vi "load cells.vi"() -> ()   [LabVIEW 2019]
doc: "The myRIO Project template acquires acceleration data from the onboard accelerometer and displays the changes of acceleration values in a waveform chart."
uses:
  <vilib>/myRIO/Instrument Drivers/Onboard IO/AI/typedefs/AI Reference.ctl
  <vilib>/myRIO/Common/Instrument Driver Framework/Utilities/typedefs/myRIO Generic Hardware Reference.ctl
  <vilib>/myRIO/Common/Instrument Driver Framework/Utilities/typedefs/Hardware Version Enum.ctl
  <vilib>/myRIO/Common/Instrument Driver Framework/Utilities/typedefs/myRIO v1.0 Reference.ctl
  <vilib>/myRIO/Common/Instrument Driver Framework/Utilities/typedefs/Generic FPGA Reference.ctl
  <vilib>/myRIO/Common/Instrument Driver Framework/myRIO v1.0/AI/typedefs/AI Channels List.ctl
  <vilib>/myRIO/Common/Instrument Driver Framework/myRIO v1.0/AI/typedefs/AI Channels Enum.ctl
  <vilib>/myRIO/Common/Instrument Driver Framework/Utilities/typedefs/Analog Scaling Constants List.ctl
  <vilib>/myRIO/Common/Instrument Driver Framework/Utilities/typedefs/Analog Scaling Constants.ctl
  <vilib>/userDefined/High Color/nirio_resource_hc.ctl
  <vilib>/myRIO/Instrument Drivers/Onboard IO/PWM/typedefs/PWM Reference.ctl
  <vilib>/myRIO/Common/Instrument Driver Framework/myRIO v1.0/PWM/typedefs/PWM Channels Enum.ctl
  <vilib>/myRIO/Instrument Drivers/Onboard IO/PWM/typedefs/PWM Configuration.ctl
  <vilib>/myRIO/Common/Instrument Driver Framework/Utilities/vis/Is FPGA Ref Available.vi
  <vilib>/myRIO/Common/Instrument Driver Framework/myRIO v1.0/AI/vis/myRIO v1.1 Open AI.vi
  <vilib>/myRIO/Instrument Drivers/Onboard IO/AI/vis/Read.vi
  <vilib>/myRIO/Common/Instrument Driver Framework/myRIO v1.0/PWM/vis/myRIO v1.1 Open PWM.vi
  <vilib>/myRIO/Common/Instrument Driver Framework/Utilities/vis/Validate Channels.vi
  <vilib>/myRIO/Common/Instrument Driver Framework/myRIO v1.0/AI/vis/myRIO v1.0 Reserve AI.vi
  <vilib>/myRIO/Common/Instrument Driver Framework/myRIO v1.0/PWM/vis/myRIO v1.0 Reserve PWM.vi
  <vilib>/myRIO/Common/Instrument Driver Framework/myRIO v1.0/PWM/vis/myRIO v1.0 Close PWM.vi
  <vilib>/myRIO/Common/Instrument Driver Framework/myRIO v1.0/AI/vis/myRIO v1.0 Build MUX Configuration AI.vi
  <vilib>/myRIO/Common/Instrument Driver Framework/myRIO v1.0/Resource Manager/vis/myRIO v1.0 Reserve Channel List.vi
  <vilib>/myRIO/Common/Instrument Driver Framework/myRIO v1.0/PWM/vis/myRIO v1.0 Build MUX Configuration PWM.vi
  <vilib>/myRIO/Common/Instrument Driver Framework/myRIO v1.0/PWM/vis/myRIO v1.0 Unreserve PWM.vi
  <vilib>/myRIO/Common/Instrument Driver Framework/myRIO v1.0/Resource Manager/vis/myRIO v1.0 Reserve Channel.vi
  <vilib>/myRIO/Common/Instrument Driver Framework/myRIO v1.0/Resource Manager/vis/myRIO v1.0 Unreserve Channel.vi
  <vilib>/myRIO/Common/Instrument Driver Framework/myRIO v1.0/Resource Manager/vis/myRIO v1.0 Create Configuration List.vi
  <vilib>/myRIO/Common/Instrument Driver Framework/myRIO v1.0/Resource Manager/vis/myRIO v1.0 Unreserve Channel List.vi
  <vilib>/myRIO/Common/Instrument Driver Framework/myRIO v1.0/Resource Manager/vis/myRIO v1.0 Build Mutex Name.vi
  <vilib>/Utility/VariantDataType/GetNumericInfo.vi
  <vilib>/Utility/error.llb/Error Cluster From Error Code.vi
  <vilib>/myRIO/Common/Instrument Driver Framework/myRIO v1.0/myRIO v1.1 Open.vi
  <vilib>/myRIO/Common/Instrument Driver Framework/myRIO v1.0/AI/vis/myRIO v1.0 Get Scaling Constants AI.vi
  <vilib>/myRIO/Common/Instrument Driver Framework/Utilities/vis/IO Manager.vi
  <vilib>/myRIO/Common/Instrument Driver Framework/Utilities/vis/Configuration Manager.vi
  <vilib>/myRIO/Common/Instrument Driver Framework/myRIO v1.0/myRIO v1.0 Close.vi
  <vilib>/myRIO/Common/Instrument Driver Framework/myRIO v1.0/AI/vis/myRIO v1.0 Read AI.vi
  <vilib>/myRIO/Common/Instrument Driver Framework/myRIO v1.0/Resource Manager/vis/myRIO v1.0 Configure IO.vi
  <vilib>/myRIO/Common/Instrument Driver Framework/myRIO v1.0/PWM/vis/myRIO v1.0 Write PWM.vi
  <vilib>/myRIO/Common/Instrument Driver Framework/myRIO v1.0/PWM/vis/myRIO v1.0 Shutdown PWM.vi
  <vilib>/myRIO/Express VI/Onboard IO/AI/AI Express VI.xnode
  <vilib>/myRIO/Instrument Drivers/Onboard IO/AI/vis/myRIO AI Open.xnode
  <vilib>/myRIO/Instrument Drivers/Onboard IO/PWM/vis/myRIO PWM Open.xnode
  <vilib>/Waveform/WDTFileIO.llb/ Write Waveform to File.vi
  <vilib>/myRIO/Instrument Drivers/Onboard IO/PWM/PWM.lvlib
  <vilib>/myRIO/Instrument Drivers/Onboard IO/AI/AI.lvlib
  <vilib>/ptbypt/NI_PtbyPt.lvlib
panel:
  out "Sum Right":dbl
  out "sum left":dbl
  out "a0":dbl format="%0.2f"
  out "appended array":dbl[](array[numeric])
  in  "cal1 3":dbl[](array[numeric])
  out "x*y 3":dbl[](array[numeric])
  out "Sensor Axial Right":T1(graph)
  out "Sensor Axial Left":T1(graph)
  in  "gain":dbl
  out "Sensor 12":dbl format="%0.2f"
  out "Sensor 10":dbl format="%0.2f"
  out "x*y 2":dbl[](array[numeric])
  in  "cal1 2":dbl[](array[numeric])
  out "Right cp2":cluster{dbl[], dbl[]}(graph)
  out "CENTER OF PRESSURE RIGHT BELT 3":dbl(graph)
  out "Sensor 8":dbl format="%0.5f"
  out "Sensor 7":dbl format="%0.5f"
  out "Sensor 6":dbl format="%0.5f"
  out "Sensor 5":dbl format="%0.5f"
  out "Sensor Rear Rigth":T1(graph)
  out "Sensor Rear Left":T1(graph)
  out "Sensor Front Right":T1(graph)
  out "Sensor Front  Left":T1(graph)
  out "RIGHT BELT SENSORS IN ONE PLOT 2":T2(graph)
  out "error out 7":errorcluster
  in  "error in 6":errorcluster
  out "error out 6":errorcluster
  in  "STOP RIGHT MOTOR":bool
  in  "RIGHT MOTOR DUTY CYCLE":dbl(slide)=50.00000000000001 scale=0.0..100.0
  out "error out 4":errorcluster
  in  "STOP LEFT MOTOR":bool
  in  "LEFT MOTOR DUTY CYCLE":dbl(slide)=50.00000000000001 scale=0.0..100.0
  in  "Stop Button":bool
  in  "ZERO ALL SENSORS":bool
  out "x*y":dbl[](array[numeric])
  in  "cal1":dbl[](array[numeric])
  out "Left cp1":cluster{dbl[], dbl[]}(graph)
  out "CENTER OF PRESSURE LEFT BELT 2":dbl(graph)
  out "dt":u32(graph)
  out "Sensor 4":dbl format="%0.5f"
  out "Sensor 3":dbl format="%0.5f"
  out "Sensor 2":dbl format="%0.5f"
  out "Sensor 1":dbl=0.0038137989155123176 format="%0.5f"
  out "Sensor Rear Rigth":T1(graph)
  out "Sensor Rear Left":T1(graph)
  out "Sensor Front Right":T1(graph)
  out "Sensor Front  Left":T1(graph)
  out "LEFT BELT SENSORS IN ONE PLOT":T2(graph)
  out "error out 5":errorcluster
  in  "error in 5":errorcluster
  # "Calibration Left"
  # "Calibration Right"
  # "Calibration Axial"
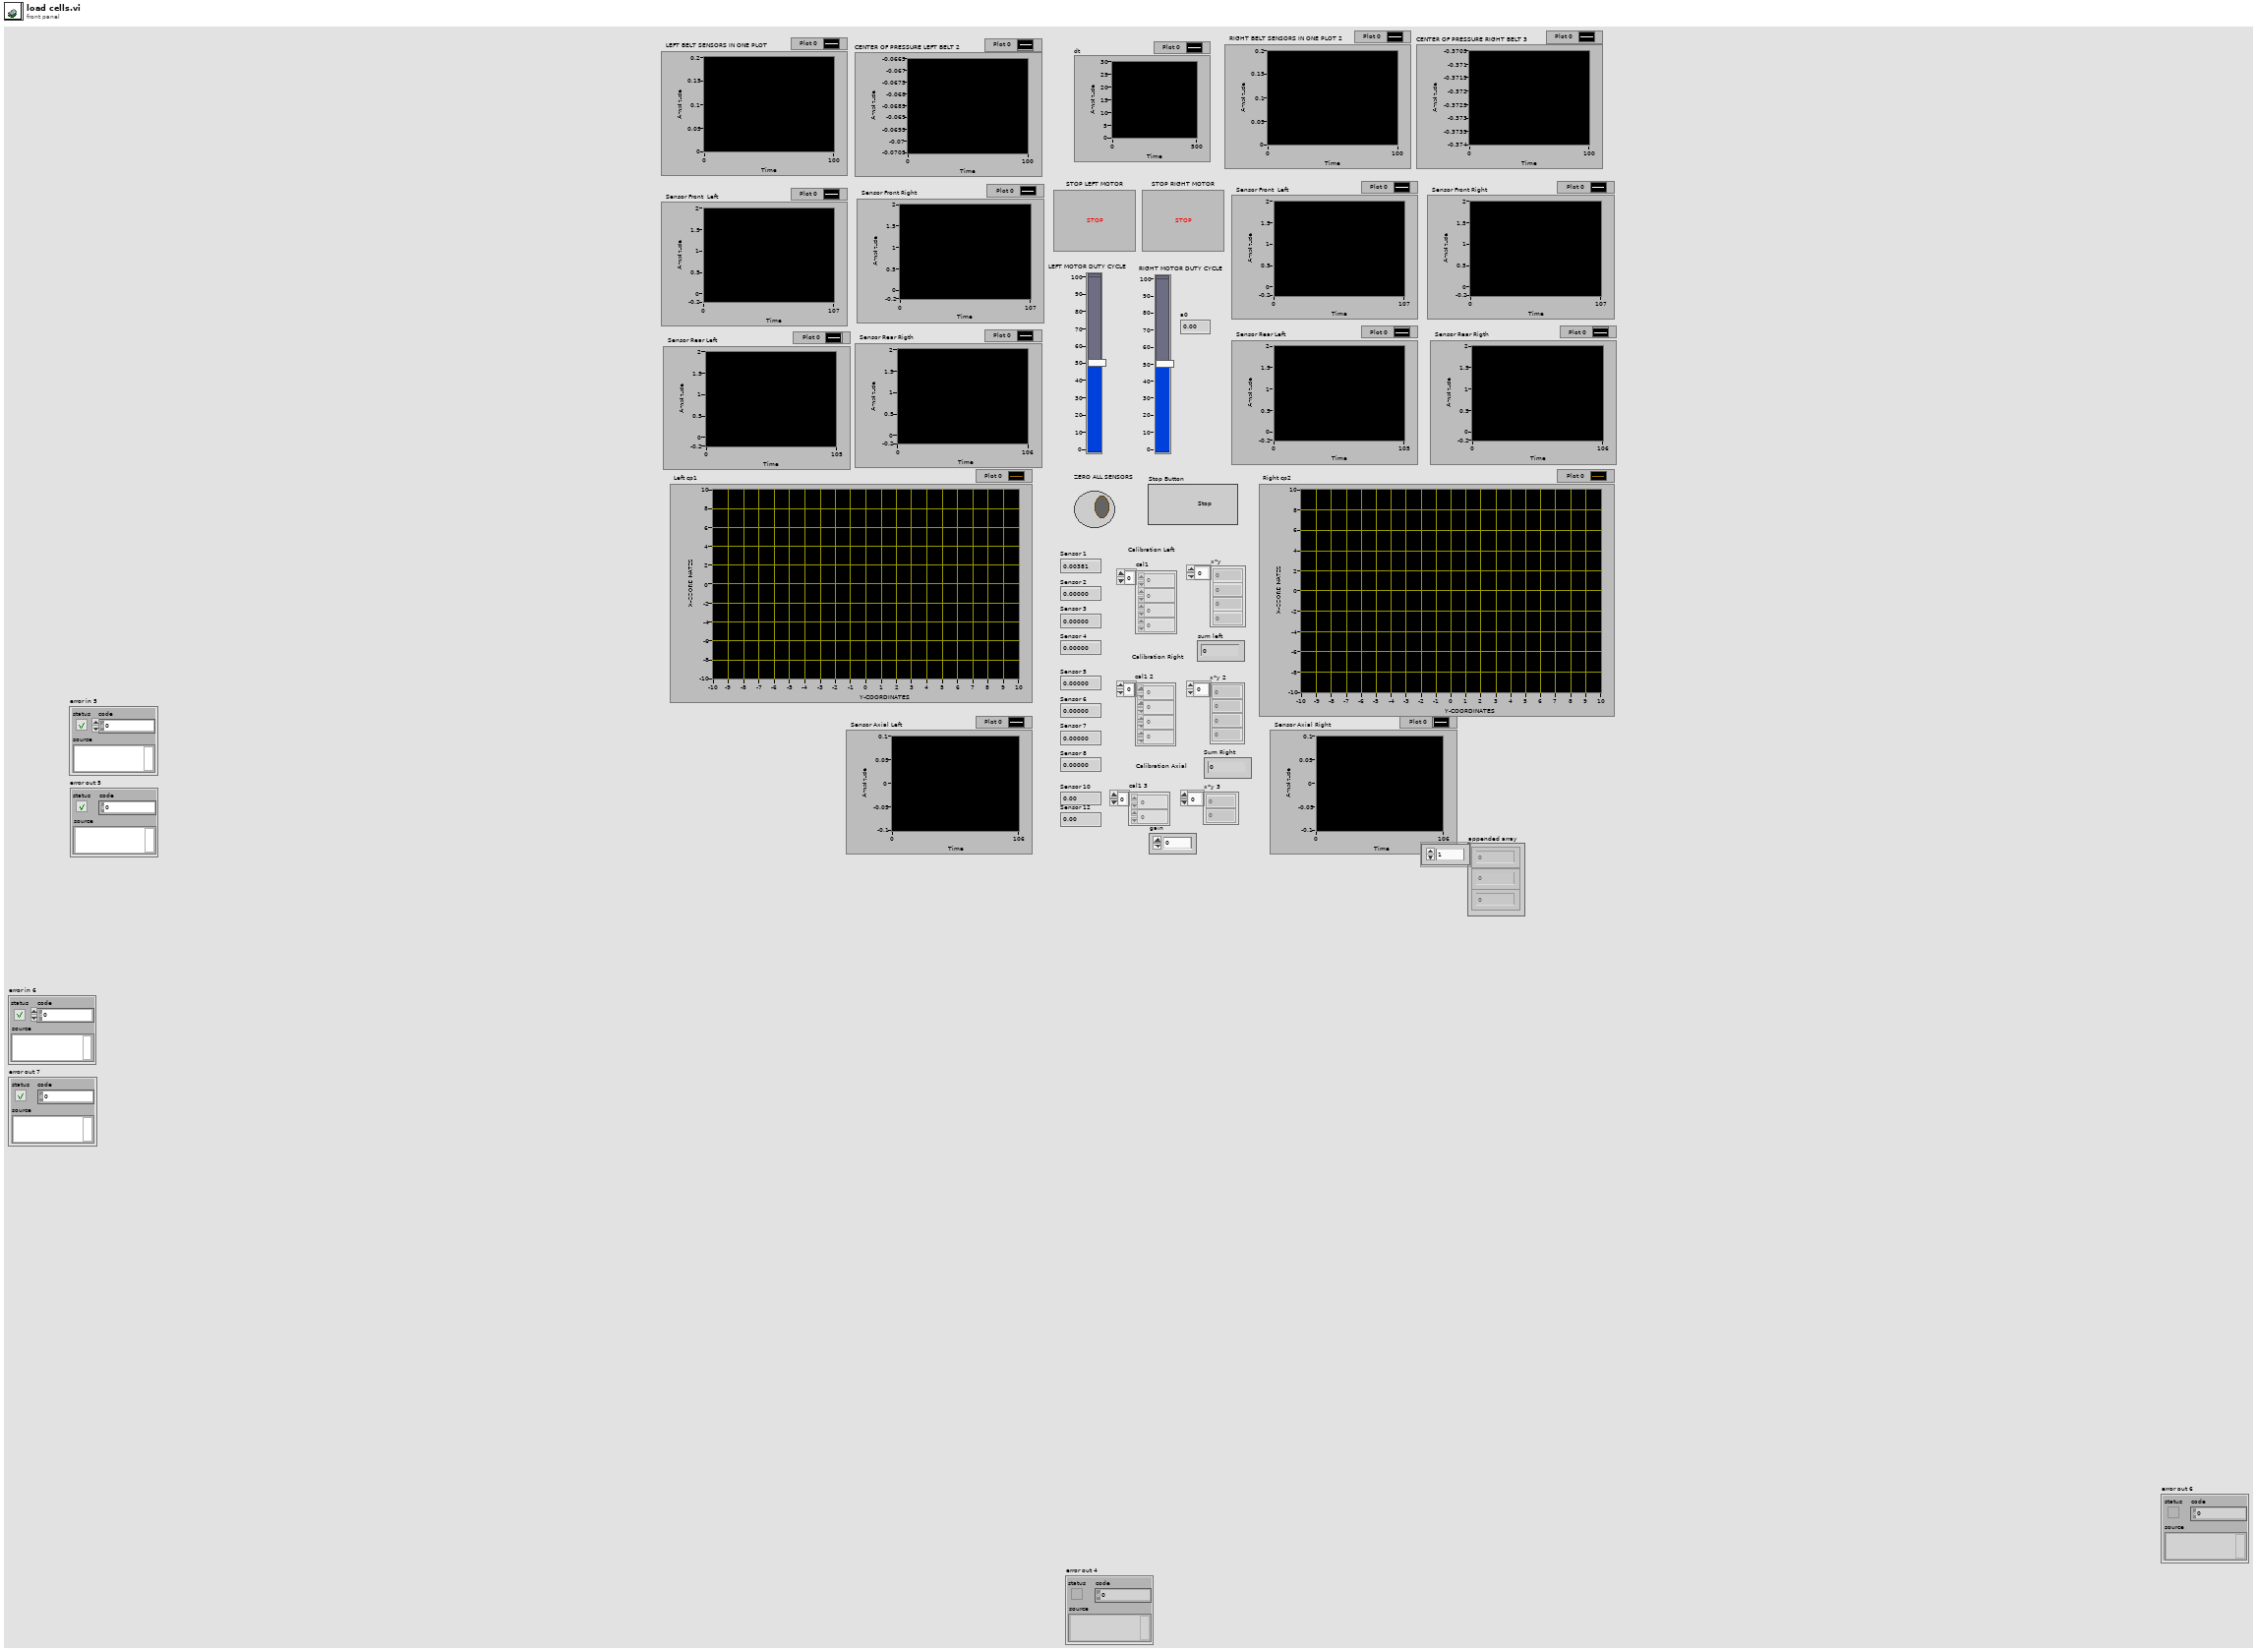
[diagram p1: front panel]
types:
  T1 = cluster{"Filtered x":dbl, "Sensor 1 (A/AI0 (Pin 3))":dbl}
  T2 = cluster{"Sensor 1 (A/AI0 (Pin 3))":dbl, "Sensor 2 (A/AI1 (Pin 5))":dbl, "Sensor 3 (A/AI2 (Pin 7))":dbl, "Sensor 4 (A/AI3 (Pin 9))":dbl}
  T3 = typedef "PWM.lvlib/PWM Reference.ctl" = cluster{"myRIO Reference":T4, "PWM Channels Enum":T8, "PWM Configuration":T9}
  T4 = typedef "myRIO Generic Hardware Reference.ctl" = cluster{"myRIO Model":T5, "myRIO Hardware Reference":T6}
  T5 = typedef "Hardware Version Enum.ctl" = enum16{"Unknown", "myRIO-1900", "myRIO-1950", "roboRIO", "NI ELVIS RIO CM", "ELVIS III"}
  T6 = typedef "myRIO v1.0 Reference.ctl" = cluster{"Generic FPGA Reference":T7, "Allow multiple opens":bool}
  T7 = typedef "Generic FPGA Reference.ctl" = refnum<k20>
  T8 = typedef "PWM Channels Enum.ctl" = enum16{"Not Connected", "C/PWM0", "C/PWM1", "A/PWM0", "A/PWM1", "A/PWM2", "A/PWM3", "A/PWM4", "A/PWM5", "A/PWM6", "A/PWM7", "A/PWM8", "A/PWM9", "A/PWM10", "A/PWM11", "A/PWM12", "A/PWM13", "A/PWM14", "A/PWM15", "A/PWM16", "A/PWM17", "A/PWM18", "A/PWM19", "B/PWM0", "B/PWM1", "B/PWM2", "B/PWM3", "B/PWM4", "B/PWM5", "B/PWM6", "B/PWM7", "B/PWM8", "B/PWM9", "B/PWM10", "B/PWM11", "B/PWM12", "B/PWM13", "B/PWM14", "B/PWM15", "B/PWM16", "B/PWM17", "B/PWM18", "B/PWM19", "PWM/PWM0", "PWM/PWM1", "PWM/PWM2", "PWM/PWM3", "PWM/PWM4", "PWM/PWM5", "PWM/PWM6", "PWM/PWM7", "PWM/PWM8", "PWM/PWM9"}
  T9 = typedef "PWM.lvlib/PWM Configuration.ctl" = cluster{"Frequency":dbl, "Duty Cycle":dbl}
  T10 = typedef "AI.lvlib/AI Reference.ctl" = cluster{"myRIO Reference":T4, "AI Channels List":T11, "AI Scaling Constants List":T13}
  T11 = typedef "AI Channels List.ctl" = T12[]
  T12 = typedef "AI Channels Enum.ctl" = enum16{"Not Connected", "AudioIn/Left", "AudioIn/Right", "C/AI0", "C/AI1", "A/AI0", "A/AI1", "A/AI2", "A/AI3", "A/AI4", "A/AI5", "A/AI6", "A/AI7", "B/AI0", "B/AI1", "B/AI2", "B/AI3", "B/AI4", "B/AI5", "B/AI6", "B/AI7", "AI/AI0", "AI/AI1", "AI/AI2", "AI/AI3", "A/AI0 (DIFF)", "A/AI1 (DIFF)", "A/AI2 (DIFF)", "A/AI3 (DIFF)", "B/AI0 (DIFF)", "B/AI1 (DIFF)", "B/AI2 (DIFF)", "B/AI3 (DIFF)"}
  T13 = typedef "Analog Scaling Constants List.ctl" = T14[]
  T14 = typedef "Analog Scaling Constants.ctl" = cluster{"LSB Weight (Volts)":dbl, "Offset (Volts)":dbl, "Signed?":bool}
  T15 = typedef "nirio_resource_hc.ctl" = tag
  T16 = cluster{"Sensor 5 (B/AI0 (Pin 3))":dbl, "Sensor 6 (B/AI1 (Pin 5))":dbl, "Sensor 7 (B/AI2 (Pin 7))":dbl, "Sensor 8 (B/AI3 (Pin 9))":dbl}
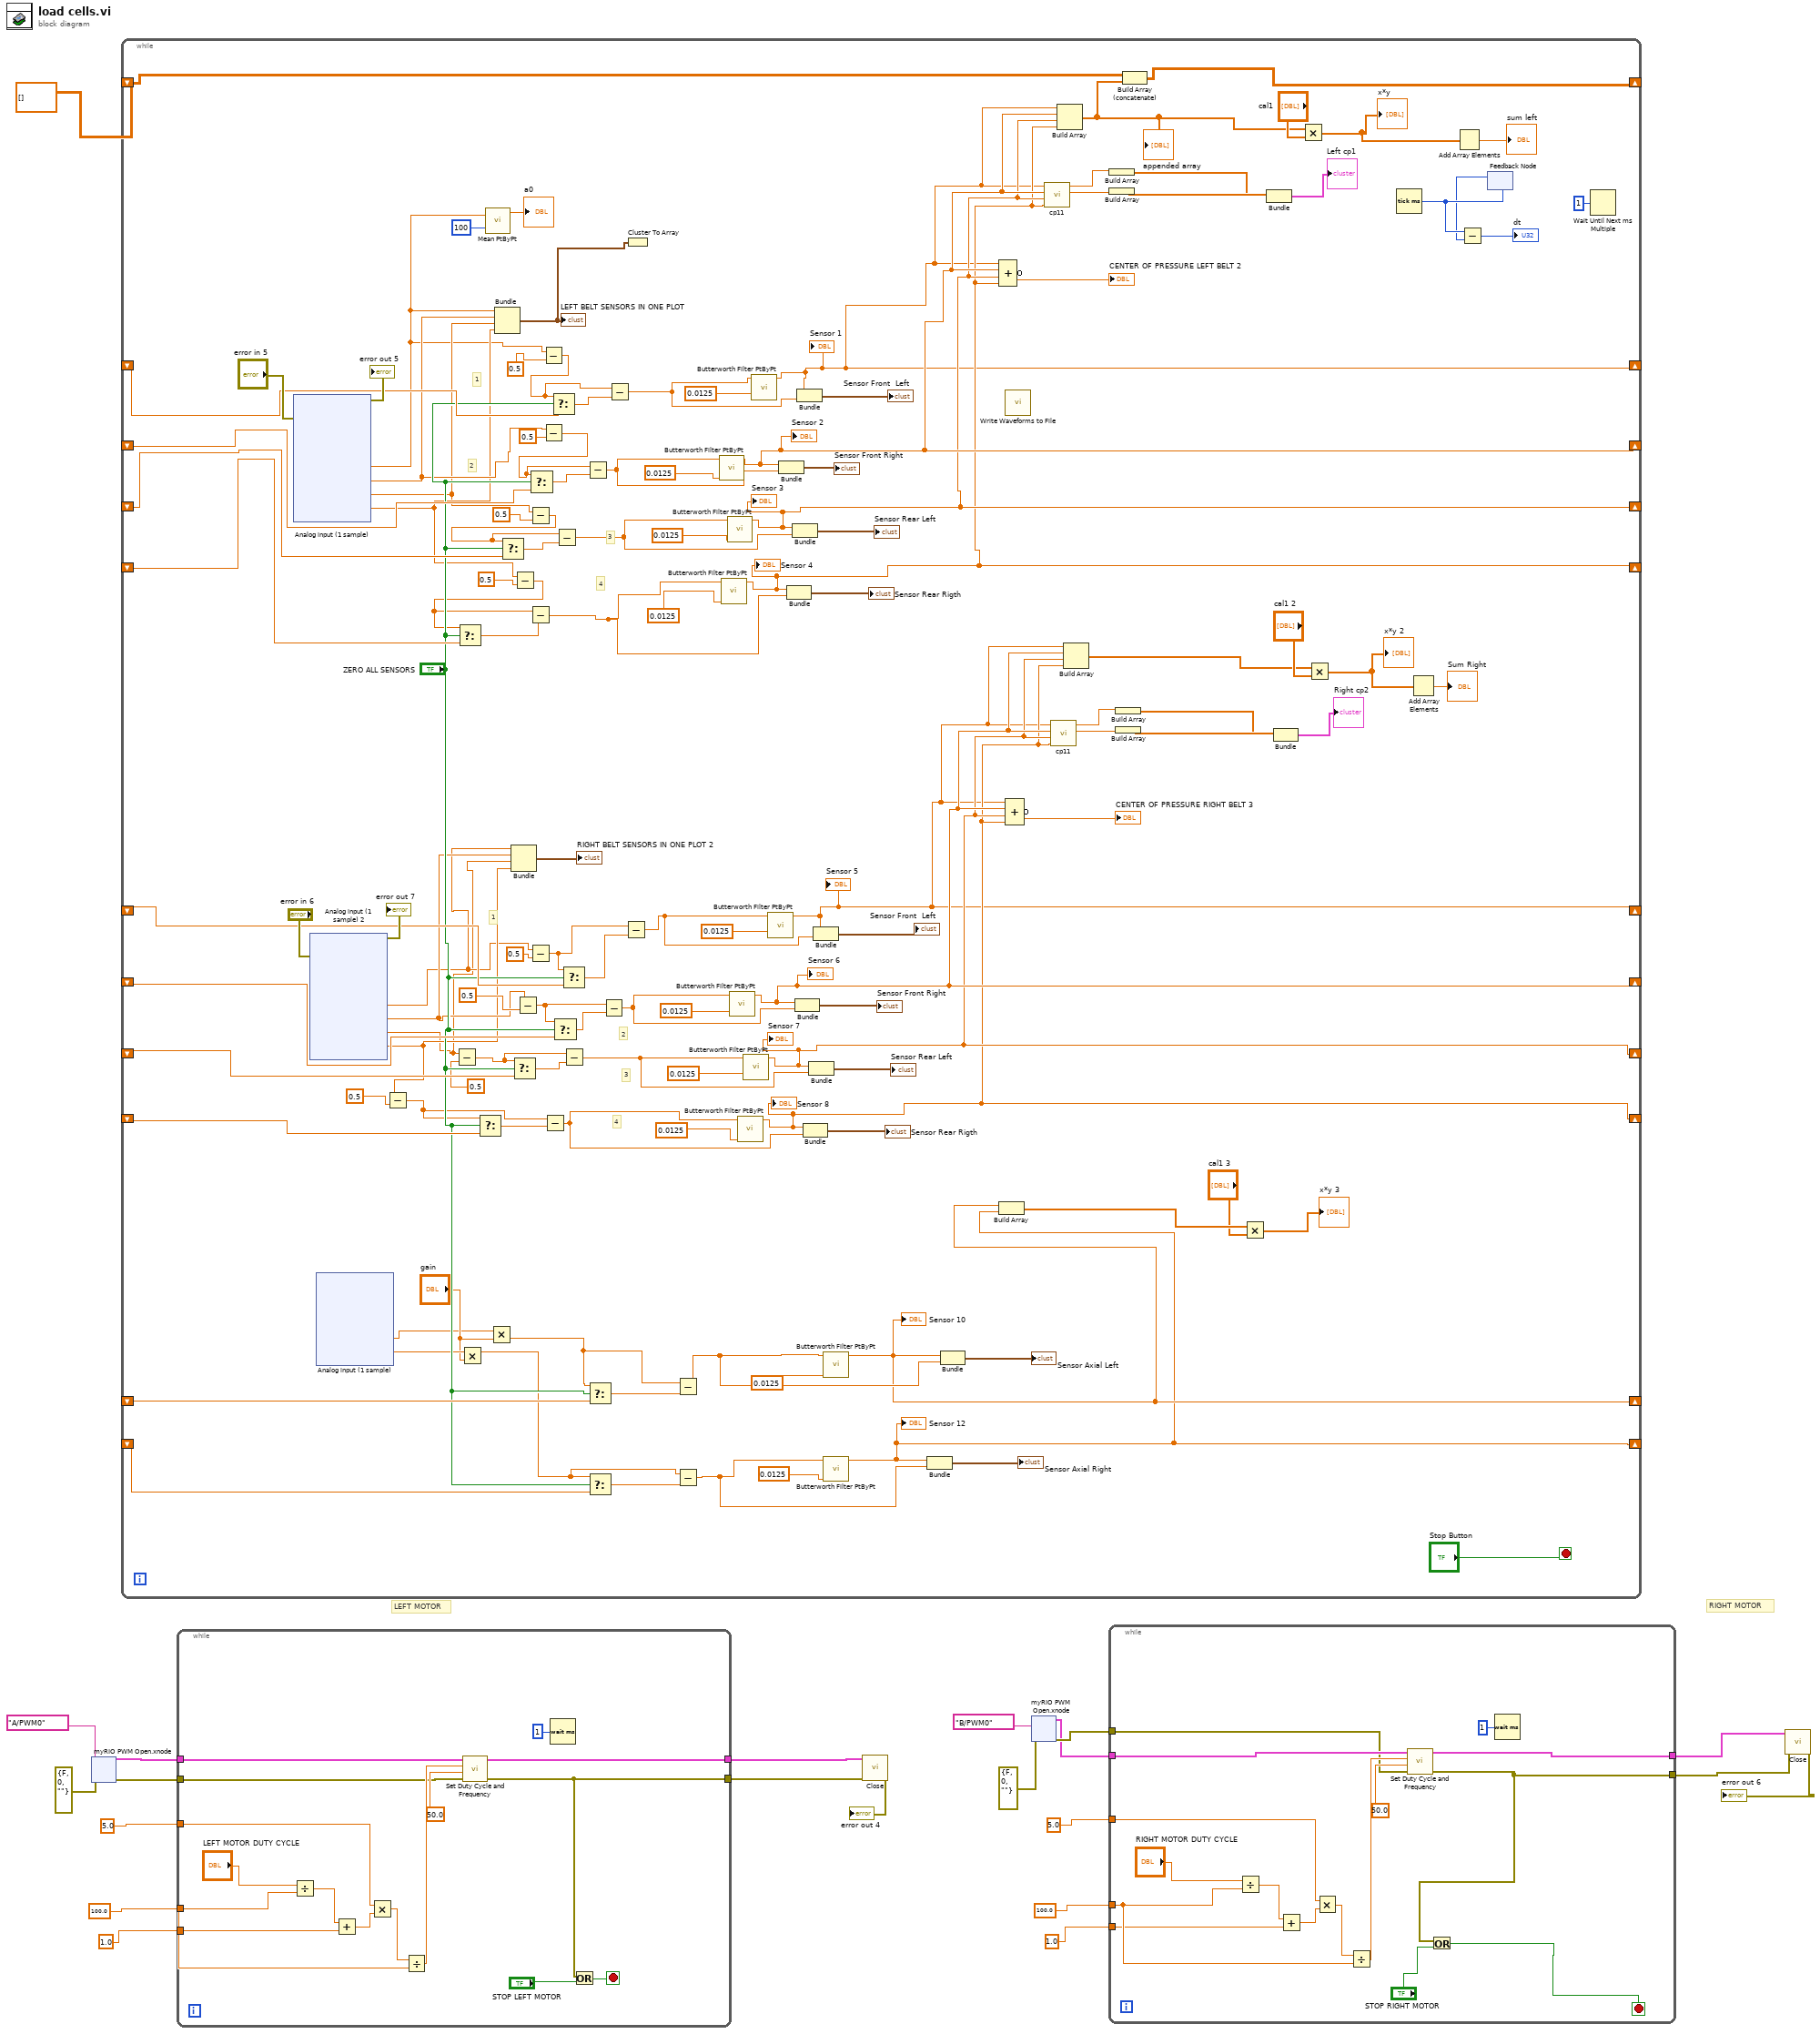
[diagram p0: block diagram]
diagram:
  # "RIGHT MOTOR"
  # "LEFT MOTOR"
  n1 = xnode "myRIO PWM Open.xnode"("error in (no error)"=errorcluster {"status"=FALSE, "code"=0, "source"=""}, "Channel Name"=tag "A/PWM0") -> ("error out"=w15:errorcluster, "PWM Ref Out"=w20:T3)  [unwired: 1 in]
  n2 = while {
    shift-right: [w44] -> _
    shift-left: _ -> [w134]
    shift-right: [w64] -> _
    shift-left: _ -> [w133]
    shift-right: [w63] -> _
    shift-left: _ -> [w132]
    shift-right: [w62] -> _
    shift-left: _ -> [w131]
    shift-right: [w61] -> _
    shift-left: _ -> [w86]
    shift-right: [w92] -> _
    shift-left: _ -> [w87]
    shift-right: [w91] -> _
    shift-left: _ -> [w88]
    shift-right: [w90] -> _
    shift-left: _ -> [w89]
    shift-right: [w66] -> _
    shift-left: _ -> [w85]
    shift-right: [w65] -> _
    shift-left: _ -> [w84]
    shift-right: [w58] -> _
    shift-left: dbl[][] [] -> [w57]
    stop <- "Stop Button" stop-if-true
    # "4"
    # "3"
    # "2"
    # "1"
    # "4"
    # "3"
    # "2"
    # "1"
    n3 = xnode "Analog input (1 sample)"("error in (no error)"="error in 5") -> ("Sensor 1 (A/AI0 (Pin 3))"=w42:dbl, "Sensor 2 (A/AI1 (Pin 5))"=w53:dbl, "Sensor 3 (A/AI2 (Pin 7))"=w47:dbl, "Sensor 4 (A/AI3 (Pin 9))"=w50:dbl, "error out"=→"error out 5":errorcluster)
    n4 = xnode "Analog input (1 sample) 2"("error in (no error)"="error in 6") -> ("Sensor 5 (B/AI0 (Pin 3))"=w27:dbl, "Sensor 6 (B/AI1 (Pin 5))"=w35:dbl, "Sensor 7 (B/AI2 (Pin 7))"=w26:dbl, "Sensor 8 (B/AI3 (Pin 9))"=w30:dbl, "error out"=→"error out 7":errorcluster)
    n5 = xnode "Analog input (1 sample)"() -> ("Sensor 9 (C/AI0) (C/AI0 (AI0))"=w72:dbl, "Sensor 10 (C/AI1) (C/AI1 (AI1))"=w78:dbl)  [unwired: 1 in, 1 out]
    n6 = Subtract(x=w30, y=0.5 ("x")) -> (x-y=w29:dbl)
    n7 = Subtract(x=w26, y=0.5) -> (x-y=w32:dbl)
    n8 = Multiply(x=w78, y="gain") -> (x*y=w74:dbl)
    n9 = Select(t=w29, s="ZERO ALL SENSORS", f=w89) -> (s? t:f=w101:dbl)
    n10 = call <vilib>:"Mean PtByPt.vi"("x"=w42, "sample length"=100) -> ("mean"=→"a0":dbl)  [unwired: 2 in, 1 out]
    n11 = Multiply(x=w72, y="gain") -> (x*y=w75:dbl)
    n12 = Bundle("Sensor 1 (A/AI0 (Pin 3))"=w42, "Sensor 2 (A/AI1 (Pin 5))"=w53, "Sensor 3 (A/AI2 (Pin 7))"=w47, "Sensor 4 (A/AI3 (Pin 9))"=w50) -> (w43:T2)  [unwired: 1 in]
    "LEFT BELT SENSORS IN ONE PLOT" <- w43
    n13 = Bundle("Sensor 5 (B/AI0 (Pin 3))"=w27, "Sensor 6 (B/AI1 (Pin 5))"=w35, "Sensor 7 (B/AI2 (Pin 7))"=w26, "Sensor 8 (B/AI3 (Pin 9))"=w30) -> (→"RIGHT BELT SENSORS IN ONE PLOT 2":T16)  [unwired: 1 in]
    n14 = Select(t=w32, s="ZERO ALL SENSORS", f=w88) -> (s? t:f=w102:dbl)
    n15 = Subtract(x=w50, y=0.5 ("Sensor 3 (A/AI2 (Pin 7))")) -> (x-y=w49:dbl)
    n16 = Select(t=w49, s="ZERO ALL SENSORS", f=w131) -> (s? t:f=w136:dbl)
    n17 = Subtract(x=w35, y=0.5 ("x")) -> (x-y=w34:dbl)
    n18 = Subtract(x=w47, y=0.5 ("Sensor 3 (A/AI2 (Pin 7))")) -> (x-y=w46:dbl)
    n19 = Select(t=w46, s="ZERO ALL SENSORS", f=w132) -> (s? t:f=w137:dbl)
    n20 = Subtract(x=w49, y=w136) -> (x-y=w39:dbl)
    n21 = Subtract(x=w27, y=0.5) -> (x-y=w28:dbl)
    n22 = Subtract(x=w42, y=0.5) -> (x-y=w59:dbl)
    n23 = Subtract(x=w53, y=0.5 ("Sensor 2 (A/AI1 (Pin 5))")) -> (x-y=w54:dbl)
    n24 = Select(t=w54, s="ZERO ALL SENSORS", f=w133) -> (s? t:f=w139:dbl)
    n25 = Subtract(x=w29, y=w101) -> (x-y=w103:dbl)
    n26 = Select(t=w59, s="ZERO ALL SENSORS", f=w134) -> (s? t:f=w141:dbl)
    n27 = Select(t=w34, s="ZERO ALL SENSORS", f=w87) -> (s? t:f=w105:dbl)
    n28 = Subtract(x=w46, y=w137) -> (x-y=w138:dbl)
    n29 = Select(t=w28, s="ZERO ALL SENSORS", f=w86) -> (s? t:f=w107:dbl)
    n30 = Subtract(x=w32, y=w102) -> (x-y=w104:dbl)
    n31 = Subtract(x=w54, y=w139) -> (x-y=w140:dbl)
    n32 = Select(t=w75, s="ZERO ALL SENSORS", f=w85) -> (s? t:f=w82:dbl)
    n33 = Select(t=w74, s="ZERO ALL SENSORS", f=w84) -> (s? t:f=w79:dbl)
    n34 = Subtract(x=w34, y=w105) -> (x-y=w106:dbl)
    n35 = Subtract(x=w59, y=w141) -> (x-y=w38:dbl)
    n36 = Subtract(x=w28, y=w107) -> (x-y=w108:dbl)
    n37 = Cluster To Array(cluster=w43) -> ()  [unwired: 1 out]
    n38 = Subtract(x=w75, y=w82) -> (x-y=w80:dbl)
    n39 = Subtract(x=w74, y=w79) -> (x-y=w76:dbl)
    n40 = call <vilib>:"Butterworth Filter PtByPt.vi"("low cutoff freq: fl"=0.0125 ("low cutoff freq: 2"), "x"=w140) -> ("Filtered x"=w64:dbl)  [unwired: 7 in, 1 out]
    "Sensor 2" <- w64
    n41 = call <vilib>:"Butterworth Filter PtByPt.vi"("low cutoff freq: fl"=0.0125 ("low cutoff freq: 4"), "x"=w39) -> ("Filtered x"=w62:dbl)  [unwired: 7 in, 1 out]
    "Sensor 4" <- w62
    n42 = call <vilib>:"Butterworth Filter PtByPt.vi"("low cutoff freq: fl"=0.0125 ("low cutoff freq: 3"), "x"=w138) -> ("Filtered x"=w63:dbl)  [unwired: 7 in, 1 out]
    "Sensor 3" <- w63
    n43 = call <vilib>:"Butterworth Filter PtByPt.vi"("low cutoff freq: fl"=0.0125 ("low cutoff freq: 2"), "x"=w106) -> ("Filtered x"=w92:dbl)  [unwired: 7 in, 1 out]
    "Sensor 6" <- w92
    n44 = call <vilib>:"Butterworth Filter PtByPt.vi"("low cutoff freq: fl"=0.0125 ("low cutoff freq: 4"), "x"=w103) -> ("Filtered x"=w90:dbl)  [unwired: 7 in, 1 out]
    "Sensor 8" <- w90
    n45 = call <vilib>:"Butterworth Filter PtByPt.vi"("low cutoff freq: fl"=0.0125 ("low cutoff freq: 3"), "x"=w104) -> ("Filtered x"=w91:dbl)  [unwired: 7 in, 1 out]
    "Sensor 7" <- w91
    n46 = call <vilib>:"Butterworth Filter PtByPt.vi"("low cutoff freq: fl"=0.0125 ("low cutoff freq: 1"), "x"=w38) -> ("Filtered x"=w44:dbl)  [unwired: 7 in, 1 out]
    "Sensor 1" <- w44
    n47 = call <vilib>:"Butterworth Filter PtByPt.vi"("low cutoff freq: fl"=0.0125 ("low cutoff freq: 1"), "x"=w108) -> ("Filtered x"=w61:dbl)  [unwired: 7 in, 1 out]
    "Sensor 5" <- w61
    n48 = Bundle("Filtered x"=w64, w140) -> (→"Sensor Front Right":cluster{"Filtered x":dbl, dbl})  [unwired: 1 in]
    n49 = Bundle("Filtered x"=w62, w39) -> (→"Sensor Rear Rigth":cluster{"Filtered x":dbl, dbl})  [unwired: 1 in]
    n50 = Bundle("Filtered x"=w63, w138) -> (→"Sensor Rear Left":cluster{"Filtered x":dbl, dbl})  [unwired: 1 in]
    n51 = Bundle("Filtered x"=w92, w106) -> (→"Sensor Front Right":cluster{"Filtered x":dbl, dbl})  [unwired: 1 in]
    n52 = Bundle("Filtered x"=w44, w38) -> (→"Sensor Front  Left":cluster{"Filtered x":dbl, dbl})  [unwired: 1 in]
    n53 = Bundle("Filtered x"=w90, w103) -> (→"Sensor Rear Rigth":cluster{"Filtered x":dbl, dbl})  [unwired: 1 in]
    n54 = Bundle("Filtered x"=w91, w104) -> (→"Sensor Rear Left":cluster{"Filtered x":dbl, dbl})  [unwired: 1 in]
    n55 = Bundle("Filtered x"=w61, w108) -> (→"Sensor Front  Left":cluster{"Filtered x":dbl, dbl})  [unwired: 1 in]
    n56 = call <vilib>:"Butterworth Filter PtByPt.vi"("low cutoff freq: fl"=0.0125 ("low cutoff freq: 4"), "x"=w80) -> ("Filtered x"=w66:dbl)  [unwired: 7 in, 1 out]
    "Sensor 10" <- w66
    n57 = call <vilib>:"Butterworth Filter PtByPt.vi"("low cutoff freq: fl"=0.0125 ("low cutoff freq: 4"), "x"=w76) -> ("Filtered x"=w65:dbl)  [unwired: 7 in, 1 out]
    "Sensor 12" <- w65
    n58 = Bundle("Filtered x"=w65, w76) -> (→"Sensor Axial Right":cluster{"Filtered x":dbl, dbl})  [unwired: 1 in]
    n59 = Bundle("Filtered x"=w66, w80) -> (→"Sensor Axial Left":cluster{"Filtered x":dbl, dbl})  [unwired: 1 in]
    n60 = Compound Arithmetic op=ADD(w44, w64, w63, w62) -> (invert →"CENTER OF PRESSURE LEFT BELT 2":dbl)
    n61 = Build Array(w66, w65) -> (w69:dbl[])
    n62 = call-poly <vilib>:"Write Waveforms to File.vi"() -> ()  [unwired: 10 in, 2 out]
    n63 = Compound Arithmetic op=ADD(w61, w92, w91, w90) -> (invert →"CENTER OF PRESSURE RIGHT BELT 3":dbl)
    n64 = call "cp11.vi"("Sensor 4 (A/AI3 (Pin 9))"=w62, "Sensor 3 (A/AI2 (Pin 7))"=w63, "Sensor 2 (A/AI1 (Pin 5))"=w64, "Sensor 1 (A/AI0 (Pin 3))"=w44) -> ("y"=w135:dbl, "x"=w121:dbl)  [unwired: 1 out]
    n65 = call "cp11.vi"("Sensor 4 (A/AI3 (Pin 9))"=w90, "Sensor 3 (A/AI2 (Pin 7))"=w91, "Sensor 2 (A/AI1 (Pin 5))"=w92, "Sensor 1 (A/AI0 (Pin 3))"=w61) -> ("y"=w100:dbl, "x"=w93:dbl)  [unwired: 1 out]
    n66 = Build Array(w44, w64, w63, w62) -> (w55:dbl[])
    "appended array" <- w55
    n67 = Build Array(w61, w92, w91, w90) -> (w96:dbl[])
    n68 = Build Array(w121) -> (w122:dbl[])
    n69 = Build Array(w135) -> (w123:dbl[])
    n70 = Build Array(w93) -> (w94:dbl[])
    n71 = Build Array(w100) -> (w95:dbl[])
    n72 = Build Array (concatenate)(w57, w55) -> (w58:dbl[][])
    n73 = Multiply(x=w69, y="cal1 3") -> (x*y=→"x*y 3":dbl[])
    n74 = Bundle(w122, w123) -> (→"Left cp1":cluster{dbl[], dbl[]})  [unwired: 1 in]
    n75 = Bundle(w94, w95) -> (→"Right cp2":cluster{dbl[], dbl[]})  [unwired: 1 in]
    n76 = Multiply(x=w55, y="cal1") -> (x*y=w25:dbl[])
    "x*y" <- w25
    n77 = Multiply(x=w96, y="cal1 2") -> (x*y=w23:dbl[])
    "x*y 2" <- w23
    n78 = Tick Count (ms)() -> (millisecond timer value=w129:u32)
    n79 = Add Array Elements(numeric array=w23) -> (sum=→"Sum Right":dbl)
    n80 = Add Array Elements(numeric array=w25) -> (sum=→"sum left":dbl)
    n81 = feedback #1() -> (w128:u32)  [unwired: 1 in]
    n82 = Subtract(x=w129, y=w128) -> (x-y=→"dt":u32)
    n83 = feedback-in #1(w129) -> ()
    n84 = Wait Until Next ms Multiple(millisecond multiple=u32 1) -> ()  [unwired: 1 out]
  }
  n85 = while {
    tunnel: w20 -> [w277]
    tunnel: [w276] -> w18
    tunnel: [w269] -> w17
    tunnel: w15 -> [w275]
    tunnel: 5.0 ("Numeric 2") -> [w274]
    tunnel: 100.0 ("Numeric") -> [w273]
    tunnel: 1.0 ("Numeric 3") -> [w272]
    stop <- w270 stop-if-true
    n86 = Divide(x="LEFT MOTOR DUTY CYCLE", y=w273) -> (x/y=w278:dbl)
    n87 = Add(x=w278, y=w272) -> (x+y=w279:dbl)
    n88 = Multiply(x=w274, y=w279) -> (x*y=w280:dbl)
    n89 = Divide(x=w280, y=w273) -> (x/y=w282:dbl)
    n90 = call <vilib>:"Set Duty Cycle and Frequency.vi"("error in (no error)"=w275, "Frequency [Hz]"=50.0, "Duty Cycle"=w282, "PWM Ref In"=w277) -> ("error out"=w269:errorcluster, "PWM Ref Out"=w276:T3)  [unwired: 5 in]
    n91 = Wait (ms)(milliseconds to wait=u32 1) -> ()  [unwired: 1 out]
    n92 = Or(x=w269, y="STOP LEFT MOTOR") -> (x .or. y?=w270:bool)
  }
  n93 = call <vilib>:"Close.vi"("error in (no error)"=w17, "PWM Ref In"=w18) -> ("error out"=→"error out 4":errorcluster)  [unwired: 9 in]
  n94 = xnode "myRIO PWM Open.xnode"("error in (no error)"=errorcluster {"status"=FALSE, "code"=0, "source"=""}, "Channel Name"=tag "B/PWM0") -> ("error out"=w8:errorcluster, "PWM Ref Out"=w3:T3)  [unwired: 1 in]
  n95 = while {
    tunnel: w3 -> [w293]
    tunnel: [w292] -> w5
    tunnel: [w284] -> w6
    tunnel: w8 -> [w291]
    tunnel: 5.0 ("Numeric 2") -> [w290]
    tunnel: 100.0 ("Numeric") -> [w289]
    tunnel: 1.0 ("Numeric 3") -> [w288]
    stop <- w285 stop-if-true
    n96 = Divide(x="RIGHT MOTOR DUTY CYCLE", y=w289) -> (x/y=w294:dbl)
    n97 = Add(x=w294, y=w288) -> (x+y=w295:dbl)
    n98 = Multiply(x=w290, y=w295) -> (x*y=w296:dbl)
    n99 = Divide(x=w296, y=w289) -> (x/y=w298:dbl)
    n100 = call <vilib>:"Set Duty Cycle and Frequency.vi"("error in (no error)"=w291, "Frequency [Hz]"=50.0, "Duty Cycle"=w298, "PWM Ref In"=w293) -> ("error out"=w284:errorcluster, "PWM Ref Out"=w292:T3)  [unwired: 5 in]
    n101 = Or(x=w284, y="STOP RIGHT MOTOR") -> (x .or. y?=w285:bool)
    n102 = Wait (ms)(milliseconds to wait=u32 1) -> ()  [unwired: 1 out]
  }
  n103 = call <vilib>:"Close.vi"("error in (no error)"=w6, "PWM Ref In"=w5) -> ("error out"=→"error out 6":errorcluster)  [unwired: 9 in]
